vi "auth_user.vi"() -> (0 "tokenReceiver":string, 1 "User_Pass":i32[](array[numeric]), 2 "urlbodyPost":string)   [LabVIEW 2020]
uses:
  <vilib>/regexp/Match Regular Expression.xnode
panel:
  out "body_outputList 2":string[](array[string])
  out "body_outputList":string[](array[string])
  out "header_outputList":string[](array[string])
  out "amount_Users":i32
  out "usersTest":string[](array[string])
  out "url_post":string
  out "url_auth":string
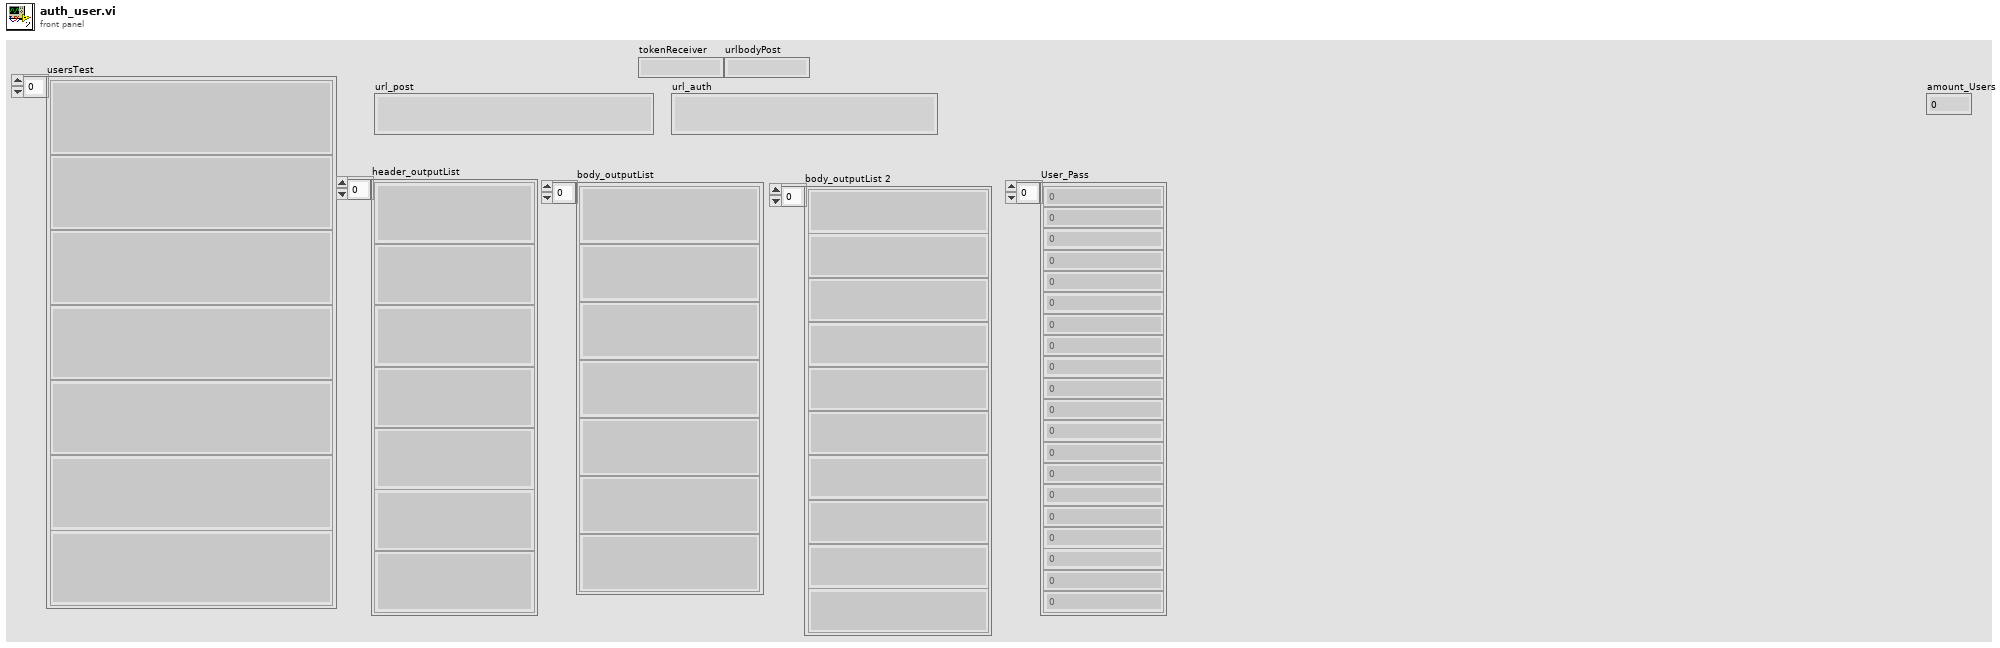
[diagram p1: front panel]
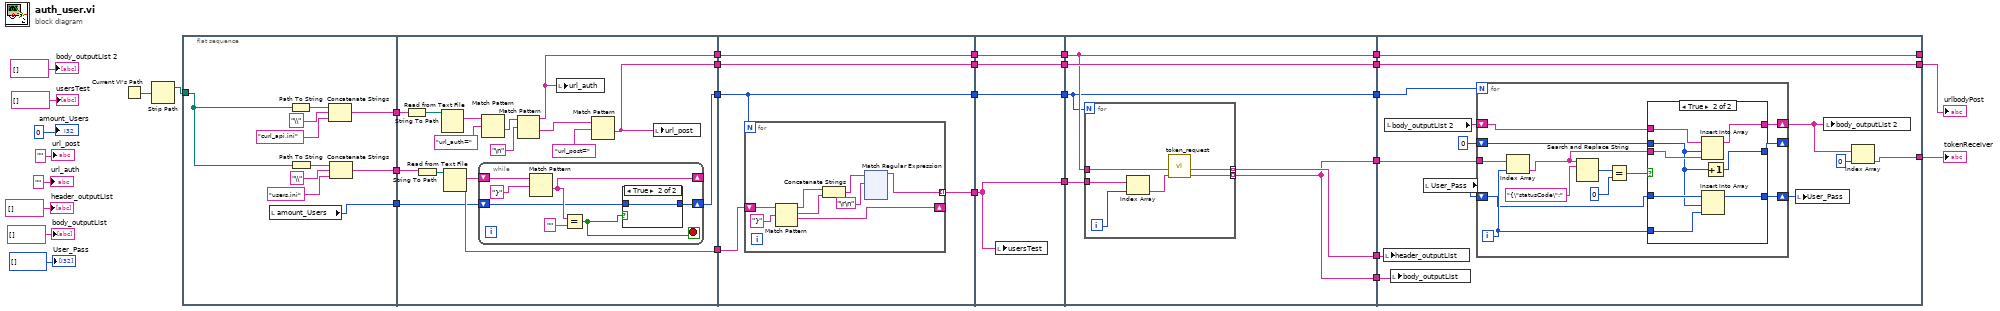
[diagram p0: block diagram]
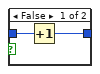
[diagram p2: hidden frame]
diagram:
  n1 = Current VI's Path() -> (path=w27:path)
  n2 = Strip Path(path=w27) -> (stripped path=w26:path)  [unwired: 1 out]
  n3 = flat-sequence {
    tunnel: [w37] -> w33
    tunnel: [w36] -> w32
    tunnel: w26 -> [w35]
    tunnel: [w34] -> w20
    tunnel: w33 -> [w58]
    tunnel: w32 -> [w51]
    tunnel: [w45] -> w31
    tunnel: [w44] -> w30
    tunnel: [w49] -> w29
    tunnel: [w48] -> w28
    tunnel: w20 -> [w46]
    tunnel: w31 -> [w70]
    tunnel: w30 -> [w71]
    tunnel: w29 -> [w69]
    tunnel: w28 -> [w73]
    tunnel: [w72] -> w25
    tunnel: [w71] -> w24
    tunnel: [w70] -> w23
    tunnel: [w69] -> w19
    tunnel: w25 -> [w196]
    tunnel: w24 -> [w199]
    tunnel: w23 -> [w198]
    tunnel: [w199] -> w22
    tunnel: [w198] -> w21
    tunnel: w19 -> [w197]
    tunnel: [w197] -> w18
    tunnel: [w196] -> w17
    tunnel: w22 -> [w203]
    tunnel: w21 -> [w205]
    tunnel: w18 -> [w200]
    tunnel: w17 -> [w204]
    tunnel: [w203] -> w16
    tunnel: [w205] -> w15
    tunnel: [w202] -> w14
    tunnel: [w201] -> w13
    tunnel: [w201] -> w12
    tunnel: [w200] -> w11
    tunnel: w16 -> [w224]
    tunnel: w15 -> [w223]
    tunnel: w14 -> [w217]
    tunnel: w13 -> [w218]
    tunnel: w12 -> [w222]
    tunnel: w11 -> [w221]
    tunnel: [w224] -> _
    tunnel: [w223] -> w1
    tunnel: [w212] -> w2
    frame #0 {
      n4 = local read "amount_Users"() -> (w34:i32)
      n5 = Path To String(path=w35) -> (string=w43:string)
      n6 = Path To String(path=w35) -> (string=w40:string)
      n7 = Concatenate Strings(w43, "\\" ("string"), "curl_api.ini" ("string")) -> (w37:string)
      n8 = Concatenate Strings(w40, "\\" ("string"), "users.ini" ("string")) -> (w36:string)
    }
    frame #1 {
      n9 = String To Path(string=w58) -> (path=w57:path)
      n10 = String To Path(string=w51) -> (path=w50:path)
      n11 = Read from Text File(file (use dialog)=w57) -> (text=w56:string)  [unwired: 3 in, 3 out]
      n12 = Read from Text File(file (use dialog)=w50) -> (text=w48:string)  [unwired: 3 in, 3 out]
      n13 = while {
        shift-right: [w63] -> _
        shift-left: w48 -> [w64]
        shift-right: [w59] -> w49
        shift-left: w46 -> [w60]
        stop <- w61 stop-if-true
        n14 = Match Pattern(string=w64, regular expression="}" ("search string")) -> (after substring=w63:string)  [unwired: 1 in, 3 out]
        n15 = Equal?(x=w63, y="") -> (x = y?=w61:bool)
        n16 = case shown="True" w61 {
          tunnel: w60 -> [w67 w68]
          tunnel: [w66 w68] -> w59
          frame False {
            n17 = Increment(x=w67) -> (x+1=w66:i32)
          }
          frame True {
          }
        }
      }
      n18 = Match Pattern(string=w56, regular expression="url_auth=") -> (after substring=w54:string)  [unwired: 1 in, 3 out]
      n19 = Match Pattern(string=w54, regular expression="\n") -> (before substring=w44:string, after substring=w53:string)  [unwired: 1 in, 2 out]
      n20 = local write "url_auth"(w44) -> ()
      n21 = Match Pattern(string=w53, regular expression="url_post=") -> (after substring=w45:string)  [unwired: 1 in, 3 out]
      n22 = local write "url_post"(w45) -> ()
    }
    frame #2 {
      n23 = for {
        N: w69 -> [_]
        shift-right: [w80] -> _
        shift-left: w73 -> [w81]
        tunnel: [w74] -> w72 mode=indexing
        n24 = Match Pattern(string=w81, regular expression="}") -> (before substring=w78:string, match substring=w77:string, after substring=w80:string)  [unwired: 1 in, 1 out]
        n25 = Concatenate Strings(w78, w77) -> (w76:string)
        n26 = xnode "Match Regular Expression"("input string"=w76, "regular expression"="\r\n") -> ("before match"=w74:string)  [unwired: 4 in, 4 out]
      }
    }
    frame #3 {
      n27 = local write "usersTest"(w196) -> ()
    }
    frame #4 {
      n28 = for {
        N: w200 -> [_]
        tunnel: w203 -> [w211]
        tunnel: w204 -> [w210]
        tunnel: [w208] -> w202 mode=indexing
        tunnel: [w207] -> w201 mode=indexing
        i -> [w206]
        n29 = Index Array(array=w210, index=w206) -> (element=w209:string)
        n30 = call "token_request.vi"("buffer"=w209, "url_input"=w211) -> ("body_output"=w207:string, "header_output"=w208:string)  [unwired: 7 in, 1 out]
      }
    }
    frame #5 {
      n31 = local write "header_outputList"(w217) -> ()
      n32 = local read "body_outputList 2"() -> (w215:string[])
      n33 = local write "body_outputList"(w218) -> ()
      n34 = local read "User_Pass"() -> (w216:i32[])
      n35 = for {
        N: w221 -> [_]
        tunnel: w222 -> [w237]
        shift-right: [w230] -> _
        shift-left: 0 -> [w231]
        shift-right: [w229] -> w214
        shift-left: w215 -> [w228]
        shift-right: [w225] -> w219
        shift-left: w216 -> [w226]
        i -> [w227]
        n36 = Index Array(array=w237, index=w227) -> (element=w232:string)
        n37 = Search and Replace String(input string=w232, search string="{\"statusCode\":") -> (number of replacements=w235:i32)  [unwired: 6 in, 3 out]
        n38 = Equal?(x=w235, y=0) -> (x = y?=w233:bool)
        n39 = case shown="True" w233 {
          tunnel: w232 -> [_ w248]
          tunnel: w231 -> [w240 w242]
          tunnel: [w240 w247] -> w230
          tunnel: [w239 w246] -> w229
          tunnel: w228 -> [w239 w245]
          tunnel: w227 -> [_ w243]
          tunnel: w226 -> [w238 w244]
          tunnel: [w238 w241] -> w225
          frame False {
          }
          frame True {
            n40 = Insert Into Array(array=w245, index=w242, new element=w248) -> (w246:string[])
            n41 = Insert Into Array(array=w244, index=w242, new element=w243) -> (w241:i32[])
            n42 = Increment(x=w242) -> (x+1=w247:i32)
          }
        }
      }
      n43 = local write "User_Pass"(w219) -> ()
      n44 = local write "body_outputList 2"(w214) -> ()
      n45 = Index Array(array=w214, index=0) -> (element=w212:string)
    }
  }
  "amount_Users" <- 0
  "body_outputList 2" <- string[] [] ("body_outputList 2")
  "usersTest" <- string[] [] ("usersTest")
  "url_post" <- "" ("url_post")
  "url_auth" <- "" ("url_auth")
  "body_outputList" <- string[] [] ("body_outputList")
  "header_outputList" <- string[] [] ("header_outputList")
  "User_Pass" <- i32[] [] ("User_Pass")
  "tokenReceiver" <- w2
  "urlbodyPost" <- w1
